vi "DIO Limits.vi"() -> (2 "Bottom Limit":bool, 3 "Top Limit":bool)   [LabVIEW 2015]
uses:
  References/Refnums.vi
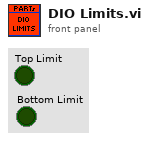
[diagram p1: front panel]
types:
  T1 = typedef "WPI_DigitalInputDevRef.ctl" = cluster{"DevStatus":errorcluster, "DIO Channel":T2}
  T2 = typedef "FPGA_DIOChannel.ctl" = enum8{"DIO 0", "DIO 1", "DIO 2", "DIO 3", "DIO 4", "DIO 5", "DIO 6", "DIO 7", "DIO 8", "DIO 9", "DIO MXP 0", "DIO MXP 1", "DIO MXP 2", "DIO MXP 3", "DIO MXP 4", "DIO MXP 5", "DIO MXP 6", "DIO MXP 7", "DIO MXP 8", "DIO MXP 9", "DIO MXP 10", "DIO MXP 11", "DIO MXP 12", "DIO MXP 13", "DIO MXP 14", "DIO MXP 15", "Invalid"}
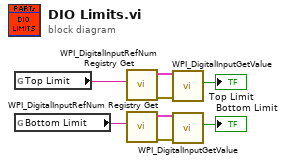
[diagram p0: block diagram]
diagram:
  n1 = global read "Refnums.vi" "Top Limit"() -> (w5:string)
  n2 = global read "Refnums.vi" "Bottom Limit"() -> (w6:string)
  n3 = call <vilib>:"WPI_DigitalInputRefNum Registry Get.vi"("refnum name"=w5) -> ("error out"=w3:errorcluster, "DigitalInputDevRef"=w4:T1)  [unwired: 9 in]
  n4 = call <vilib>:"WPI_DigitalInputRefNum Registry Get.vi"("refnum name"=w6) -> ("error out"=w8:errorcluster, "DigitalInputDevRef"=w7:T1)  [unwired: 9 in]
  n5 = call <vilib>:"WPI_DigitalInputGetValue.vi"("error in (no error)"=w3, "DigitalInputDevRef"=w4) -> ("Value"=→"Top Limit":bool)  [unwired: 7 in, 2 out]
  n6 = call <vilib>:"WPI_DigitalInputGetValue.vi"("error in (no error)"=w8, "DigitalInputDevRef"=w7) -> ("Value"=→"Bottom Limit":bool)  [unwired: 7 in, 2 out]
